vi "Pad TAB.vi"(10 "Separator":string="\t", 11 "Input String Array":string[](array[string])) -> (3 "Output String":string)   [LabVIEW 2021]
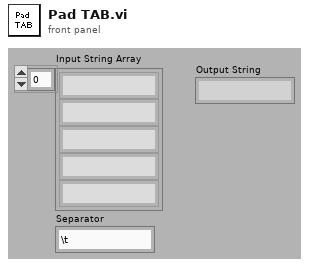
[diagram p1: front panel]
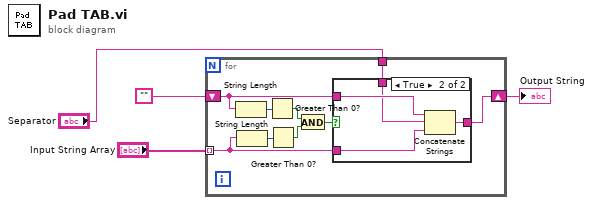
[diagram p0: block diagram]
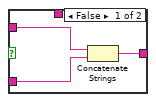
[diagram p2: hidden frame]
diagram:
  n1 = for {
    tunnel: "Input String Array" -> [w7] mode=indexing
    shift-right: [w6] -> w2
    shift-left: "" -> [w8]
    tunnel: "Separator" -> [w5]
    n2 = String Length(string=w8) -> (length=w13:i32)
    n3 = String Length(string=w7) -> (length=w12:i32)
    n4 = Greater Than 0?(x=w13) -> (x > 0?=w10:bool)
    n5 = Greater Than 0?(x=w12) -> (x > 0?=w11:bool)
    n6 = And(x=w10, y=w11) -> (x .and. y?=w9:bool)
    n7 = case shown="True" w9 {
      tunnel: w8 -> [w15 w19]
      tunnel: [w16 w20] -> w6
      tunnel: w7 -> [w14 w18]
      tunnel: w5 -> [_ w17]
      frame False {
        n8 = Concatenate Strings(w15, w14) -> (w16:string)
      }
      frame True {
        n9 = Concatenate Strings(w19, w17, w18) -> (w20:string)
      }
    }
  }
  "Output String" <- w2
